vi "Read PowerData.vi"(8 "error in (no error)":errorcluster, 11 "SetPower Message":refnum<class "SetPower Message.lvclass">) -> (0 "error out":errorcluster, 2 "PowerData":T1, 3 "SetPower Message":refnum<class "SetPower Message.lvclass">)   [LabVIEW 2018, in "QMH_Class.lvlib" / "TestManager.lvlib" / "SetPower Message.lvclass"]
uses:
  SetPower Message.lvclass
  SetPower Message.lvclass/SetPower Message.ctl
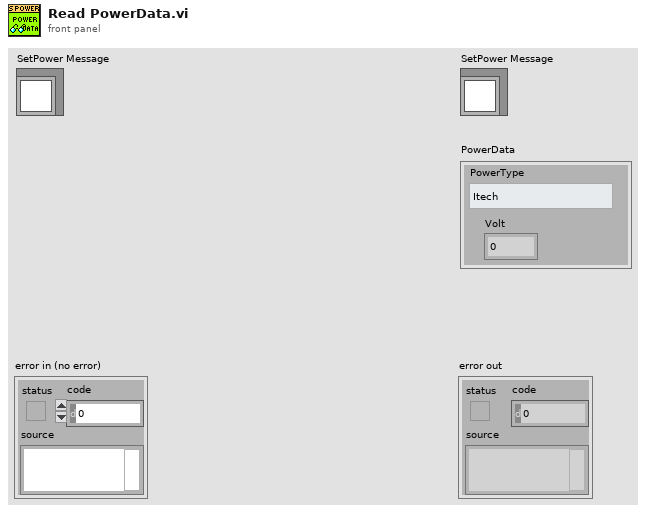
[diagram p1: front panel]
types:
  T1 = cluster{"Volt":dbl, "PowerType":enum16{"Itech", "Keysight"}}
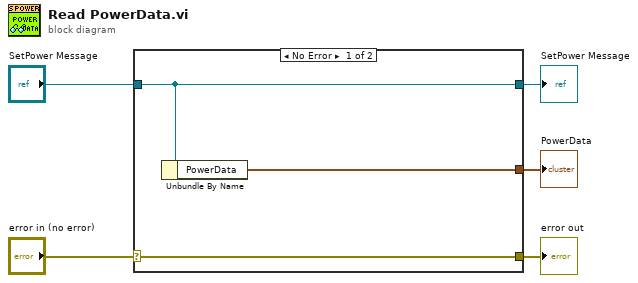
[diagram p0: block diagram]
diagram:
  n1 = case shown="No Error" "error in (no error)" {
    selector: "error in (no error)" -> [w8 w9]
    tunnel: [w8 w9] -> w4
    tunnel: [w7 w10] -> w2
    tunnel: "SetPower Message" -> [w7 w10]
    tunnel: [w6 _] -> w1
    frame No Error {
      n2 = Unbundle By Name(w7) -> ("PowerData"=w6:T1)
    }
    frame Error {
    }
  }
  "error out" <- w4
  "SetPower Message" <- w2
  "PowerData" <- w1
